vi "Password.vi"() -> (0 "Cancel":bool)   [LabVIEW 2009]
panel:
  in  "Cancel Button":bool
  in  "OK Button":bool
  in  "Password":string caption="Please enter maintenance password:"
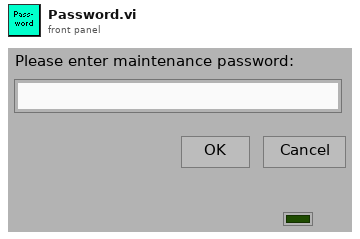
[diagram p1: front panel]
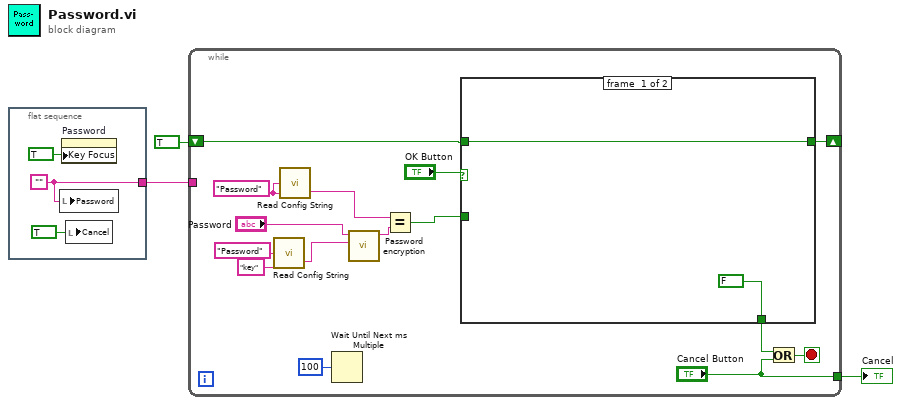
[diagram p0: block diagram]
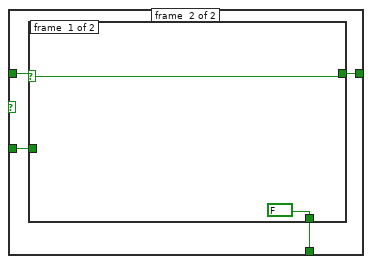
[diagram p2: hidden frame]
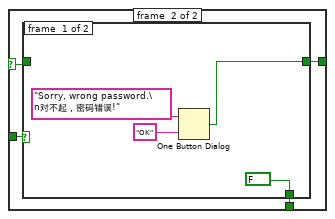
[diagram p3: hidden frame]
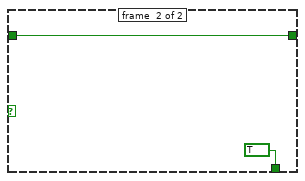
[diagram p4: hidden frame]
diagram:
  n1 = flat-sequence {
    tunnel: [w6] -> w3
    frame #0 {
      w6 = ""
      n2 = local write "Password"(w6) -> ()
      n3 = property on="Password" class="String"("Key Focus"=TRUE) -> ()  [unwired: 2 in, 2 out]
      n4 = local write "Cancel"(TRUE ("Cancel")) -> ()
    }
  }
  n5 = while {
    tunnel: w3 -> [_]
    tunnel: ["Cancel Button"] -> w2
    shift-right: [w14] -> _
    shift-left: TRUE -> [w13]
    stop <- w17 stop-if-true
    w11 = "Password" ("section")
    n6 = call "Read Config String.vi"("key"="key", "section"="Password") -> ("String"=w8:string)  [unwired: 1 in, 1 out]
    n7 = call "Read Config String.vi"("key"=w11, "section"=w11) -> ("String"=w7:string)  [unwired: 1 in, 1 out]
    n8 = Wait Until Next ms Multiple(millisecond multiple=u32 100) -> ()  [unwired: 1 out]
    n9 = call "Password encryption.vi"("Key"=w8, "Password"="Password") -> ("Output text"=w20:string)  [unwired: 1 in, 6 out]
    n10 = Equal?(x=w7, y=w20) -> (x = y?=w18:bool)
    n11 = case shown="True" "OK Button" {
      tunnel: w18 -> [_ w27]
      tunnel: [FALSE w26] -> w16
      tunnel: w13 -> [w22 w24]
      tunnel: [w22 w25] -> w14
      frame #0 {
      }
      frame #1 {
        n12 = case shown="True" w24 {
          selector: w24 -> [w29 w30]
          tunnel: w27 -> [_ w33]
          tunnel: [FALSE w32] -> w26
          tunnel: [w29 w31] -> w25
          frame #0 {
          }
          frame #1 {
            n13 = case shown="False" w33 {
              tunnel: [FALSE TRUE] -> w32
              tunnel: w30 -> [_ w38]
              tunnel: [w34 w38] -> w31
              frame #0 {
                n14 = One Button Dialog(message="Sorry, wrong password.\n对不起，密码错误!", button name ("OK")="OK" ("T button name (\"OK\")")) -> (true=w34:bool)
              }
              frame #1 {
              }
            }
          }
        }
      }
    }
    n15 = Or(x=w16, y="Cancel Button") -> (x .or. y?=w17:bool)
  }
  "Cancel" <- w2
